vi "createSALCommand.vi"(8 "error in":errorcluster, 10 "CommandID":dbl, 11 "Command.lvclass":refnum<class "Command.lvclass">) -> (0 "error out":errorcluster, 3 "SALCommand.lvclass out":refnum<class "SALCommand.lvclass">)   [LabVIEW 2016, in "SALCommand.lvclass"]
uses:
  SALCommand.lvclass
  ComponentTemplateCore/ComponentModel/ComponentModel/Command/Command.lvclass
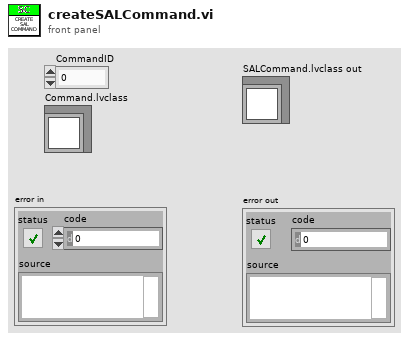
[diagram p1: front panel]
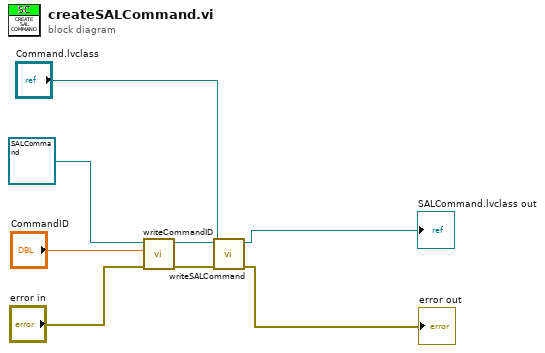
[diagram p0: block diagram]
diagram:
  n1 = call "writeCommandID.vi"("error in"="error in", "CommandID"="CommandID", "SALCommand.lvclass in"=refnum<class "SALCommand.lvclass"> refnum) -> ("error out"=w5:errorcluster, "SALCommand.lvclass out"=w7:refnum<class "SALCommand.lvclass">)  [unwired: 7 in]
  n2 = call "writeSALCommand.vi"("error in"=w5, "Command.lvclass"="Command.lvclass", "SALCommand.lvclass in"=w7) -> ("error out"=→"error out":errorcluster, "SALCommand.lvclass out"=→"SALCommand.lvclass out":refnum<class "SALCommand.lvclass">)  [unwired: 7 in]
